vi "scaler_analog_12channels_example.vi"() -> ()   [LabVIEW 2017]
uses:
  <vilib>/Platform/TimedLoop/XDataNode/timing_clust.ctl
  <vilib>/Platform/TimedLoop/XDataNode/nitl_modes.ctl
  <vilib>/Platform/TimedLoop/XDataNode/wakeup.ctl
  <vilib>/rvi/Emulation/niFpgaGetClockAttributes.vi
  <vilib>/rvi/Emulation/niFpgaSctlEmulationGetInTimedLoop.vi
  <vilib>/rvi/Emulation/niFpgaEmulationReportErrorSimple.vi
  <vilib>/rvi/Emulation/niFpgaCriticalErrorInLSC.vi
  <vilib>/rvi/Emulation/niFpgaProcessEmulError.vi
  <vilib>/rvi/eio/common/nirviEmuTemplateMethod_errors.vi
  <vilib>/Platform/TimedLoop/XDataNode/XDataNode.xnode
  <vilib>/eio/EIONode/EIONode.xnode
  lib/Scaler-EPICS/scaler.lvlib
  <vilib>/Platform/TimedLoop/XDataNode/XDNodeRunTimeDep.lvlib
panel:
  out "Looptime":u32
  in  "sample":bool
  out "Done_Scaler":bool
  out "Counter_Scaler":u32[](array[numeric])
  in  "Enable_Scaler":bool
  in  "OneShot_Scaler":bool
  in  "Gate_Scaler":bool[](array[boolean])=[FALSE, FALSE, FALSE, FALSE, FALSE, FALSE, FALSE, FALSE, FALSE, FALSE, FALSE, FALSE]
  in  "PresetValues_Scaler":u32[](array[numeric])=[0, 0, 0, 0, 0, 0, 0, 0, 0, 0, 0, 0]
  in  "AnalogInputs_Scaler":u32[](array[numeric])=[0, 0, 0, 0, 0, 0, 0, 0, 0, 0, 0, 0]
  # "This is a 12 channel analog scaler. It follows to the word the definition of the scaler in the anl website\nhttps://epics.anl.gov/bcda/synApps/std/scalerRecord.html"
  # "Optimization tip:\nMake all the arrays the same size as the number\nof channels you need implemented. Setting\nthe number of channels uses up to 60% of the \nresources. Setting to 2 uses only 27%."
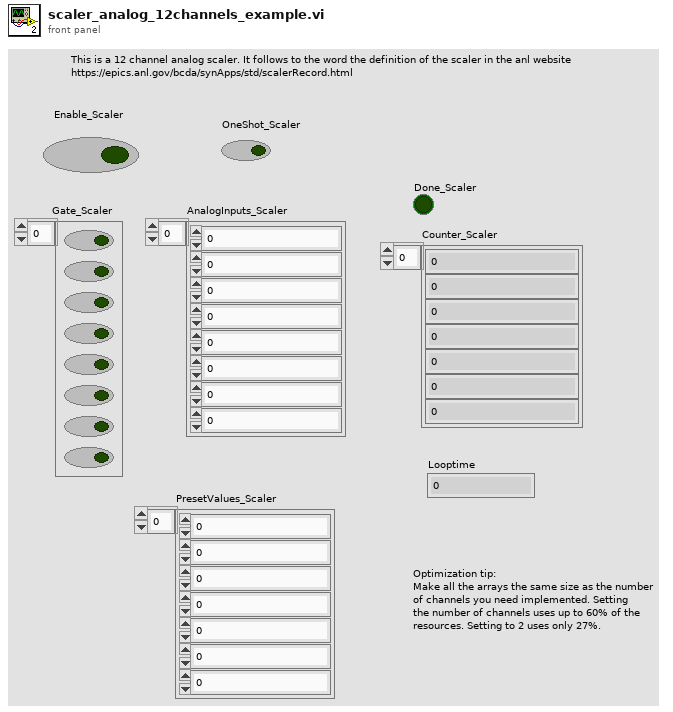
[diagram p1: front panel]
types:
  T1 = typedef "XDNodeRunTimeDep.lvlib/timing_clust.ctl" = cluster{"Expected End [f-1]":u64, "Actual End [f-1]":u64, "Finished Late? [f-1]":bool, "Expected End [i-1]":u64, "Actual End [i-1]":u64, "Finished Late? [i-1]":bool, "Expected Start [i]":u64, "Actual Start [i]":u64, "Expected Start [f]":u64, "Actual Start [f]":u64, "Source Name":string, "Structure Name":string, "Period":i64, "Deadline":i64, "Offset":i64, "Start":i64, "Priority":i32, "Timeout":i32, "Mode":T2, "Wakeup Reason":T3, "Error":errorcluster, "Source Type":string, "Secondary Source Type":string, "Global End Time":u64, "Global Start Time":u64, "Frame Duration":u64, "Iteration Duration":u64, "Assigned CPU":i32, "I/O Scan Engine Mode":u32}
  T2 = typedef "XDNodeRunTimeDep.lvlib/nitl_modes.ctl" = enum32{"No Change", "Process missed periods, maintain original phase", "Discard missed periods, maintain original phase", "Process missed periods, ignore original phase", "Discard missed periods, ignore original phase"}
  T3 = typedef "XDNodeRunTimeDep.lvlib/wakeup.ctl" = enum32{"Normal", "Aborted", "Asynchronous wakeup", "Timing source error", "Timed loop error", "Timeout"}
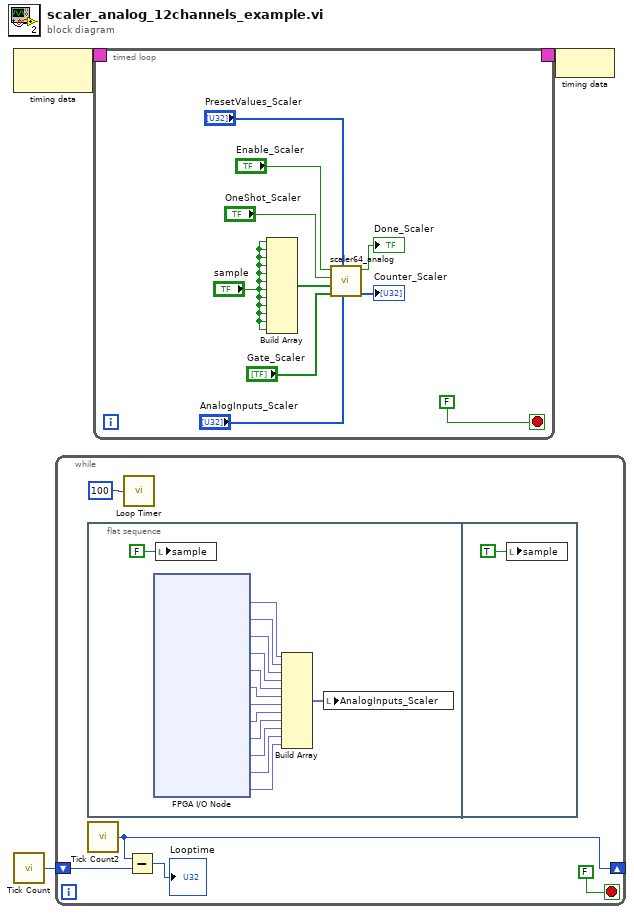
[diagram p0: block diagram]
diagram:
  n1 = node-c288() -> (w3:T1)  [unwired: 1 in]
  n2 = call "Tick Count"() -> ("Tick Count(Ticks)"=w1:u32)
  n3 = while {
    shift-right: [w5] -> _
    shift-left: w1 -> [w6]
    stop <- FALSE stop-if-true
    n4 = flat-sequence {
      frame #0 {
        n5 = xnode "FPGA I/O Node"() -> ("Mod4/AI0"=w22:fxp<+/-,20,5>, "Mod4/AI1"=w19:fxp<+/-,20,5>, "Mod4/AI2"=w18:fxp<+/-,20,5>, "Mod4/AI3"=w17:fxp<+/-,20,5>, "Mod7/AI0"=w16:fxp<+/-,20,5>, "Mod7/AI1"=w15:fxp<+/-,20,5>, "Mod7/AI2"=w14:fxp<+/-,20,5>, "Mod7/AI3"=w13:fxp<+/-,20,5>, "Mod8/AI0"=w12:fxp<+/-,20,5>, "Mod8/AI1"=w11:fxp<+/-,20,5>, "Mod8/AI2"=w10:fxp<+/-,20,5>, "Mod8/AI3"=w9:fxp<+/-,20,5>)  [unwired: 12 in, 12 out]
        n6 = local write "sample"(FALSE) -> ()
        n7 = Build Array(w22, w19, w18, w17, w16, w15, w14, w13, w12, w11, w10, w9) -> (w21:fxp<+/-,20,5>[])
        n8 = local write "AnalogInputs_Scaler"(w21) -> ()
      }
      frame #1 {
        n9 = local write "sample"(TRUE ("sample")) -> ()
      }
    }
    n10 = call "Tick Count2"() -> ("Tick Count(Ticks)"=w5:u32)
    n11 = call "Loop Timer"("Count(Ticks)"=i16 100) -> ()  [unwired: 1 out]
    n12 = Subtract(x=w5, y=w6) -> (x-y=→"Looptime":u32)
  }
  n13 = timed-loop {
    timing: w3 -> [_]
    timing-out: [_] -> w2
    stop <- FALSE stop-if-true
    n14 = Build Array("sample", "sample", "sample", "sample", "sample", "sample", "sample", "sample", "sample", "sample", "sample", "sample") -> (w25:bool[])
    n15 = call "scaler64_analog.vi"("AnalogInputs_Scaler"="AnalogInputs_Scaler", "PresetValues_Scaler"="PresetValues_Scaler", "Gate_Scaler"="Gate_Scaler", "Pulse_Scaler"=w25, "OneShot_Scaler"="OneShot_Scaler", "Enable_Scaler"="Enable_Scaler") -> ("Counter_Scaler"=→"Counter_Scaler":u32[], "Done_Scaler"=→"Done_Scaler":bool)  [unwired: 4 in]
  }
  n16 = node-c288(w2) -> ()
